vi "pruebaun solo pin varia  - copia.vi"() -> ()   [LabVIEW 2011]
uses:
  <vilib>/LabVIEW Interface for Arduino/Type Defs/Arduino Resource.ctl
  <vilib>/LabVIEW Interface for Arduino/Type Defs/Board Type.ctl
  <vilib>/LabVIEW Interface for Arduino/Type Defs/Pin Mode.ctl
  <vilib>/LabVIEW Interface for Arduino/LabVIEW Interface for Arduino.lvlib
panel:
  out "Arduino Resource":T1={"VISA resource"="", "Board Type"=enum."Uno", "Connection Type"=enum."USB / Serial", "Bytes Per Packet (15)"=15}
  out "error out":errorcluster
  in  "stop":bool
  out "x*y":u8
  out "Voltage":dbl(knob) scale=0.0..5.0
  out "PWM Pins":u8[](array[numeric])
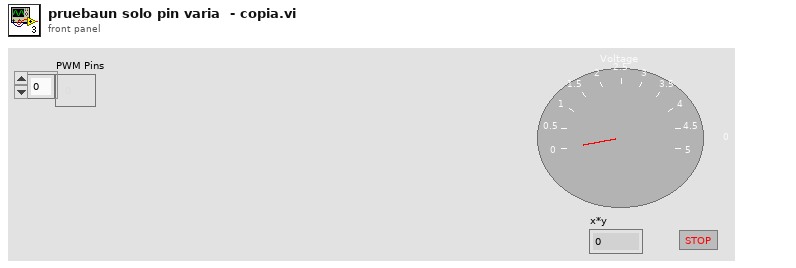
[diagram p1: front panel]
types:
  T1 = typedef "LabVIEW Interface for Arduino.lvlib/Arduino Resource.ctl" = cluster{"VISA resource":refnum<visa-resource-name>, "Board Type":T2, "Connection Type":enum8{"USB / Serial"}, "Bytes Per Packet (15)":u8}
  T2 = typedef "LabVIEW Interface for Arduino.lvlib/Board Type.ctl" = enum16{"Uno", "Dimuelanove w/Atmega 328", "Mega 2560"}
  T3 = typedef "LabVIEW Interface for Arduino.lvlib/Pin Mode.ctl" = enum8{"Input", "Output"}
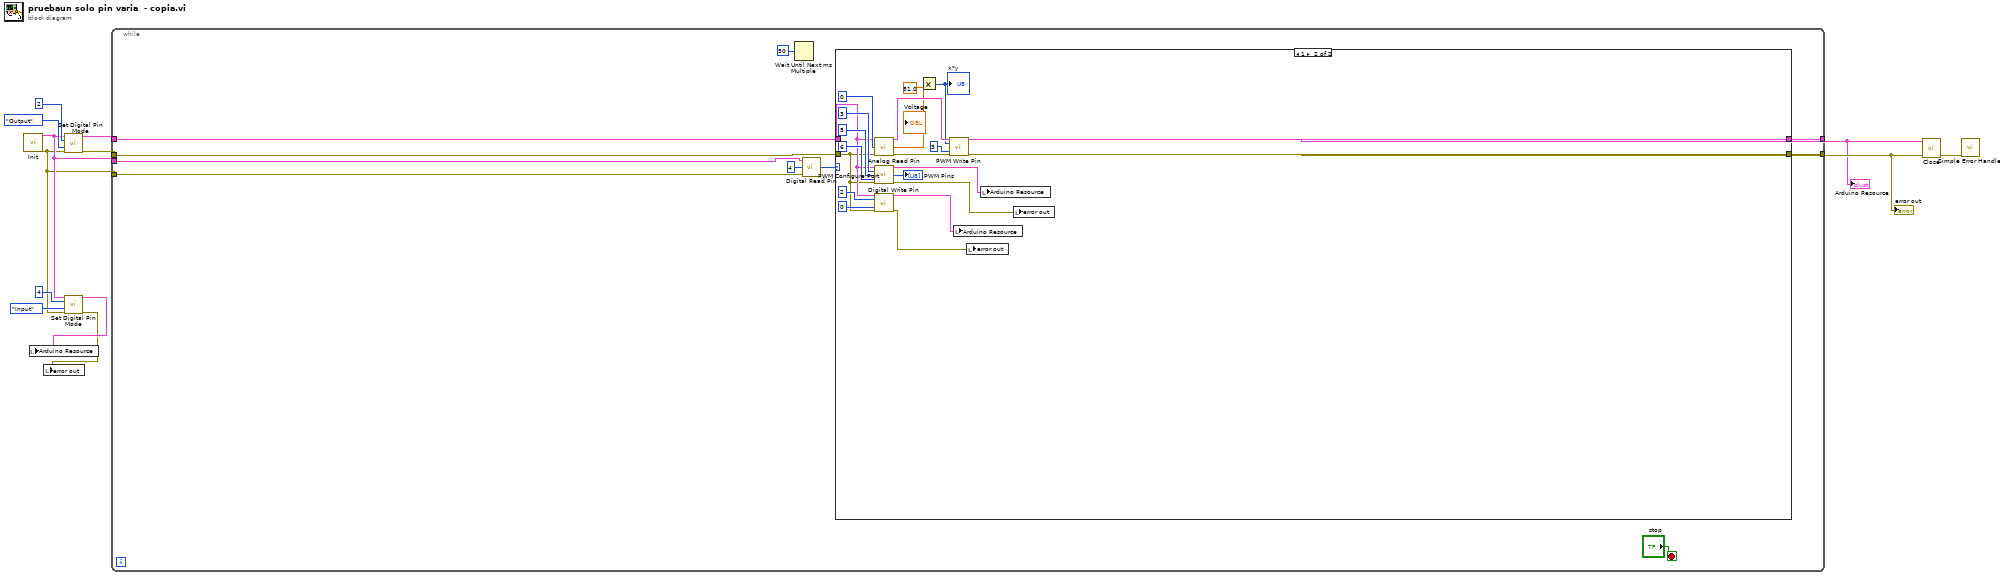
[diagram p0: block diagram]
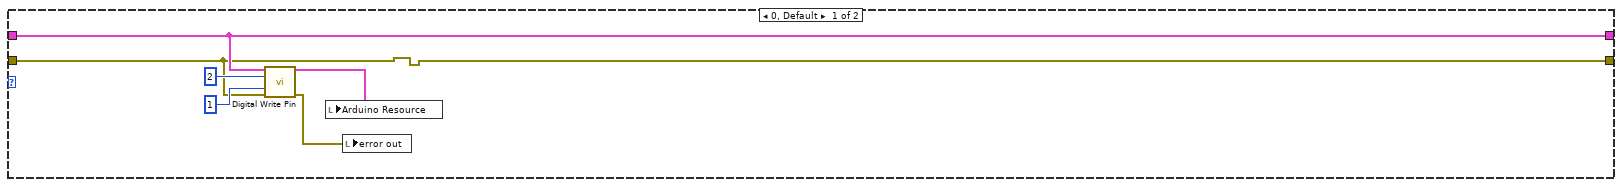
[diagram p2: hidden frame]
diagram:
  n1 = call <vilib>:"Init.vi"() -> ("Arduino Resource"=w6:T1, "error out"=w5:errorcluster)  [unwired: 18 in]
  n2 = call <vilib>:"Set Digital Pin Mode.vi"("Arduino Resource"=w6, "Digital I/O Pin"=u8 2, "Pin Mode (Input)"=Pin_Mode."Output", "error in"=w5) -> ("Arduino Resource"=w9:T1, "error out"=w8:errorcluster)  [unwired: 10 in]
  n3 = call <vilib>:"Set Digital Pin Mode.vi"("Arduino Resource"=w6, "Digital I/O Pin"=u8 4, "Pin Mode (Input)"=Pin_Mode."Input", "error in"=w5) -> ("Arduino Resource"=w4:T1, "error out"=w3:errorcluster)  [unwired: 10 in]
  n4 = local write "Arduino Resource"(w4) -> ()
  n5 = local write "error out"(w3) -> ()
  n6 = while {
    tunnel: w9 -> [w17]
    tunnel: w8 -> [w16]
    tunnel: [w23] -> w1
    tunnel: [w22] -> w2
    tunnel: w6 -> [w15]
    tunnel: w5 -> [w14]
    stop <- "stop" stop-if-true
    n7 = Wait Until Next ms Multiple(millisecond multiple=u32 50) -> ()  [unwired: 1 out]
    n8 = call <vilib>:"Digital Read Pin.vi"("Arduino Resource"=w15, "Digital I/O Pin (0)"=u8 4, "error in"=w14) -> ("Value"=w19:u8)  [unwired: 10 in, 2 out]
    n9 = case shown="1" w19 {
      tunnel: w16 -> [w26 w36]
      tunnel: w17 -> [w27 w37]
      tunnel: [w27 w40] -> w23
      tunnel: [w26 w34] -> w22
      frame 0, Default {
        n10 = call <vilib>:"Digital Write Pin.vi"("Arduino Resource"=w27, "Digital I/O Pin (0)"=u8 2, "Value (0)"=u8 1, "error in"=w26) -> ("Arduino Resource"=w25:T1, "error out"=w24:errorcluster)  [unwired: 10 in]
        n11 = local write "Arduino Resource"(w25) -> ()
        n12 = local write "error out"(w24) -> ()
      }
      frame 1 {
        n13 = call <vilib>:"Analog Read Pin.vi"("Arduino Resource"=w37, "Analog Input Pin (0)"=u8 0, "error in"=w36) -> ("Arduino Resource"=w44:T1, "Voltage"=w35:dbl, "error out"=w43:errorcluster)  [unwired: 10 in]
        "Voltage" <- w35
        n14 = call <vilib>:"PWM Configure Port.vi"("Arduino Resource"=w37, "PWM Pin (3)"=u8 3, "PWM Pin (5)"=u8 5, "PWM Pin (6)"=u8 6, "error in"=w36) -> ("Arduino Resource"=w33:T1, "PWM Pins"=→"PWM Pins":u8[], "error out"=w32:errorcluster)  [unwired: 8 in]
        n15 = call <vilib>:"Digital Write Pin.vi"("Arduino Resource"=w37, "Digital I/O Pin (0)"=u8 2, "Value (0)"=u8 0, "error in"=w36) -> ("Arduino Resource"=w31:T1, "error out"=w30:errorcluster)  [unwired: 10 in]
        n16 = Multiply(x=w35, y=51.0) -> (x*y=w41:u8)
        "x*y" <- w41
        n17 = call <vilib>:"PWM Write Pin.vi"("Arduino Resource"=w44, "Duty Cycle (0 - 255)"=w41, "PWM Pin (3)"=u8 3, "error in"=w43) -> ("Arduino Resource"=w40:T1, "error out"=w34:errorcluster)  [unwired: 10 in]
        n18 = local write "Arduino Resource"(w31) -> ()
        n19 = local write "error out"(w30) -> ()
        n20 = local write "Arduino Resource"(w33) -> ()
        n21 = local write "error out"(w32) -> ()
      }
    }
  }
  "Arduino Resource" <- w1
  "error out" <- w2
  n22 = call <vilib>:"Close.vi"("Arduino Resource"=w1, "error in"=w2) -> ("error out"=w7:errorcluster)  [unwired: 13 in]
  n23 = call <vilib>:"Simple Error Handler.vi"("error in (no error)"=w7) -> ()  [unwired: 4 in, 5 out]
